vi "Close PropToPC Port.vi"(11 "GIC Input":T1={"     Use ?\nOff       On"=[FALSE, TRUE, FALSE, TRUE], "Mode:"=FALSE, "Rx Prop Port"="", "Hokuyo Port"="COM7", "Tx Prop  Port"="COM6", "Compass Port"="", "GPS Port"="", "Num of WPs"=0, "WP Lats and Longs"={"WP Lats"=[], "WP Longs"=[]}, "Obst Lats and Longs"={"Obst Lats"=[], "Obst Longs"=[]}, "Parameters"=[], "GPS Data"=[], "Compass"=0.0, "LMS Vector"=[], "Vision Vector"=[], "Direction Cmd"=0.0, "Speed Cmd"=0.0, "WP Vector"=[], "WP Number"=0, "Extra"=0, "SW Map"=[], "Path Cluster"={"Path x node"=[], "Path y node"=[]}} {"Obst Lats and Longs"."Obst Longs" format="%#_8g"; "Obst Lats and Longs"."Obst Lats" format="%#_8g"}) -> ()   [LabVIEW 2014]
panel:
  # "Close Prop To PC Port"
  # "Input:"
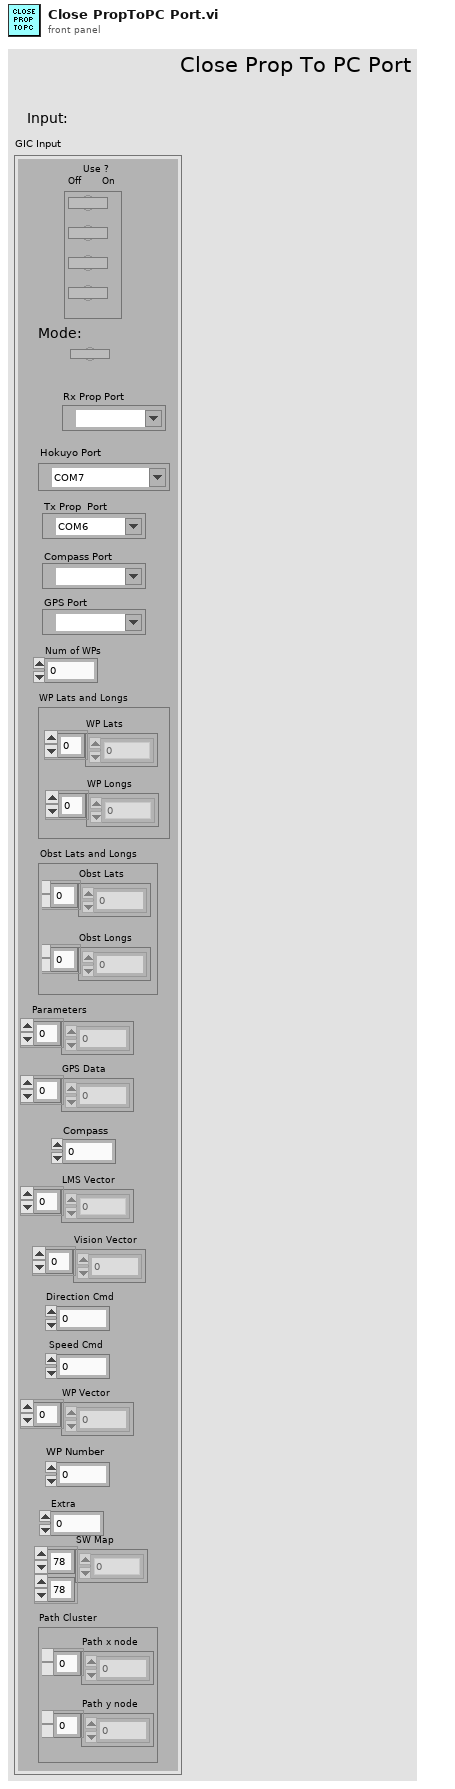
[diagram p1: front panel]
types:
  T1 = cluster{"     Use ?\nOff       On":bool[], "Mode:":bool, "Rx Prop Port":refnum<visa-resource-name>, "Hokuyo Port":refnum<visa-resource-name>, "Tx Prop  Port":refnum<visa-resource-name>, "Compass Port":refnum<visa-resource-name>, "GPS Port":refnum<visa-resource-name>, "Num of WPs":i16, "WP Lats and Longs":cluster{"WP Lats":dbl[], "WP Longs":dbl[]}, "Obst Lats and Longs":cluster{"Obst Lats":dbl[], "Obst Longs":dbl[]}, "Parameters":dbl[], "GPS Data":dbl[], "Compass":dbl, "LMS Vector":dbl[], "Vision Vector":dbl[], "Direction Cmd":dbl, "Speed Cmd":dbl, "WP Vector":dbl[], "WP Number":i32, "Extra":i16, "SW Map":i32[][], "Path Cluster":cluster{"Path x node":dbl[], "Path y node":dbl[]}}
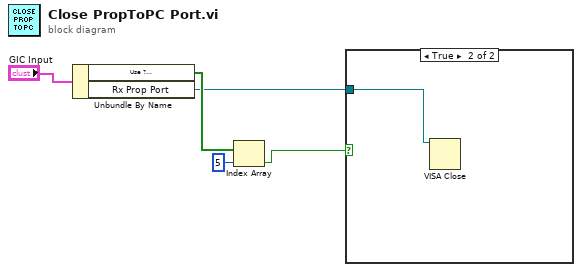
[diagram p0: block diagram]
diagram:
  n1 = Unbundle By Name("GIC Input") -> ("Use ?\nOff       On"=w4:bool[], "Rx Prop Port"=w1:refnum<visa-resource-name>)
  n2 = Index Array(array=w4, index=5) -> (element=w2:bool)
  n3 = case shown="True" w2 {
    tunnel: w1 -> [_ w6]
    frame False {
    }
    frame True {
      n4 = VISA Close(VISA resource name=w6) -> ()  [unwired: 1 in, 1 out]
    }
  }
